vi "Real Vector Norm.vi"(9 "user defined norm":dbl=-1.0, 10 "norm type":T1=2 items=["1-norm"=1, "2-norm"=2, "Inf-norm"=3, "-Inf-norm"=4, "User Defined"=5], 11 "Input Vector":dbl[](array[numeric])) -> (0 "error":i32, 3 "norm":dbl)   [LabVIEW 2020, in "NI_AALPro.lvlib"]
doc: "Computes the <B>norm</B> of <B>Input Vector</B>. Wire data to the <B>Input Vector</B> input to determine the polymorphic instance to use or manually select the instance."
uses:
  NI_AALPro.lvlib
  Vector Norm Type.ctl
  <resource>/lvanlys.dll
panel:
  # "Vector Norm"
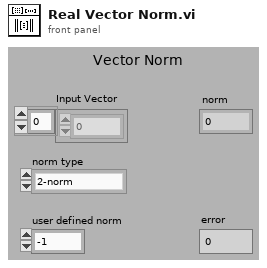
[diagram p1: front panel]
types:
  T1 = typedef "NI_AALPro.lvlib/Vector Norm Type.ctl" = u16
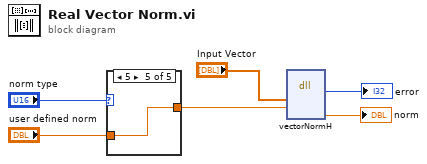
[diagram p0: block diagram]
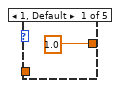
[diagram p2: hidden frame]
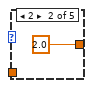
[diagram p3: hidden frame]
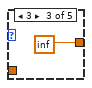
[diagram p4: hidden frame]
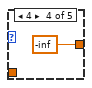
[diagram p5: hidden frame]
diagram:
  n1 = case shown="5" "norm type" {
    tunnel: [1.0 2.0 inf -inf w11] -> w2
    tunnel: "user defined norm" -> [_ _ _ _ w11]
    frame 1, Default {
    }
    frame 2 {
    }
    frame 3 {
    }
    frame 4 {
    }
    frame 5 {
    }
  }
  n2 = dll-call lib="C:/Program Files (x86)/National Instruments/LabVIEW 2020/resource/lvanlys.*" fn="vectorNormH"("xH"="Input Vector", "p"=w2) -> ("return type"=→"error":i32, "norm"=→"norm":dbl)  [unwired: 6 in, 2 out]
